vi "DPO4034 Fetch Measurement.vi"(7 "Destination Channel (1: Channel 2)":u16(ring)=1 items=["Channel 1", "Channel 2", "Channel 3", "Channel 4", "Math", "Reference 1", "Reference 2", "Reference 3", "Reference 4"], 8 "error in (no error)":errorcluster, 9 "Measurement Function (0: Period)":i32(ring) items=["Period", "Frequency", "Delay", "Rise Time", "Fall Time", "Positive Duty Cycle", "Negative Duty Cycle", "Positive Pulse Width", "Negative Pulse Width", "Burst Width", "Phase", "Positive Overshoot", "Negative Overshoot", "Vpp", "Amplitude", "Voltage High", "Voltage Low", "Voltage Max", "Voltage Min", "Voltage Mean", "Voltage Mean (cycle)", "Voltage RMS", "Voltage RMS (cycle)", "Area", "Cycle Area", "Positive Edge Count", "Negative Edge Count", "Positive Pulse Count", "Negative Pulse Count"], 10 "Channel (0: Channel 1)":u16(ring) items=["Channel 1", "Channel 2", "Channel 3", "Channel 4", "Math", "Reference 1", "Reference 2", "Reference 3", "Reference 4"], 11 "VISA resource name":refnum<visa-resource-name>) -> (0 "error out":errorcluster, 2 "Measurement Value":dbl, 3 "VISA resource name out":refnum<visa-resource-name>)   [LabVIEW 2012]
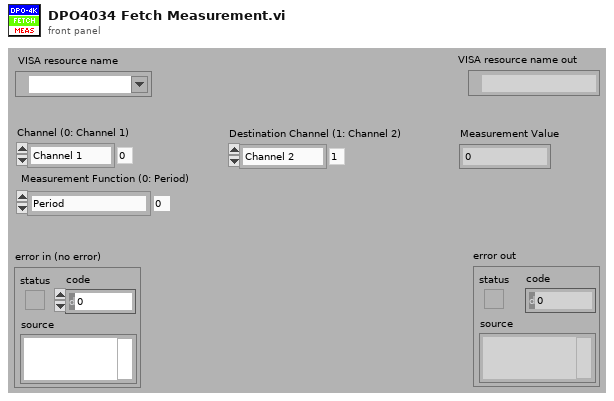
[diagram p1: front panel]
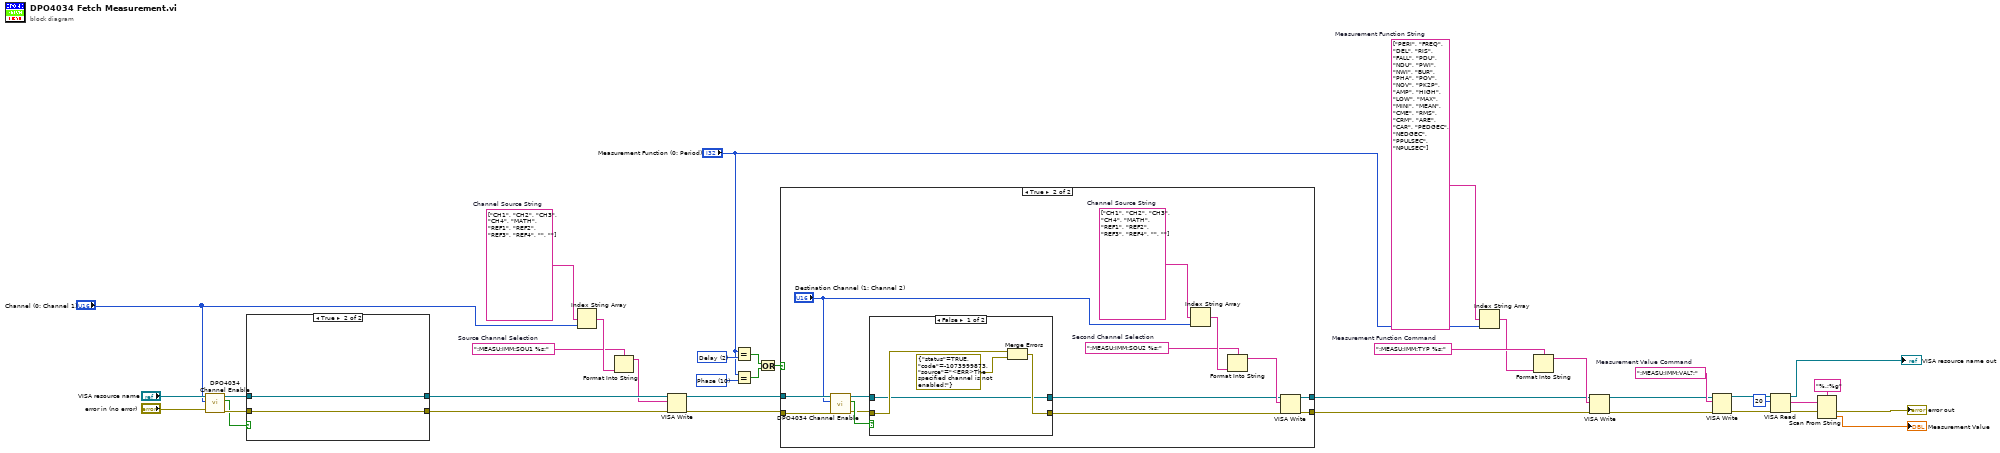
[diagram p0: block diagram]
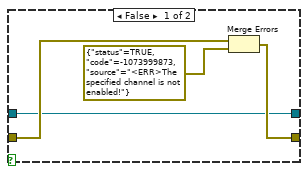
[diagram p2: hidden frame]
diagram:
  w12 = ":MEASU:IMM:SOU1 %s;"  # Source Channel Selection
  w11 = string[] ["CH1", "CH2", "CH3", "CH4", "MATH", "REF1", "REF2", "REF3", "REF4", "", ""]  # Channel Source String
  w26 = ":MEASU:IMM:VAL?;"  # Measurement Value Command
  w34 = u16 10 items=["Period", "Frequency", "Delay", "Rise Time", "Fall Time", "Positive Duty Cycle", "Negative Duty Cycle", "Positive Pulse Width", "Negative Pulse Width", "Burst Width", "Phase", "Positive Overshoot", "Negative Overshoot", "Pk-Pk", "Amplitude", "High", "Low", "Max", "Min", "Mean", "Cycle Mean", "RMS", "Cycle RMS", "Area", ""]
  w35 = u16 2 items=["Period", "Frequency", "Delay", "Rise Time", "Fall Time", "Positive Duty Cycle", "Negative Duty Cycle", "Positive Pulse Width", "Negative Pulse Width", "Burst Width", "Phase", "Positive Overshoot", "Negative Overshoot", "Pk-Pk", "Amplitude", "High", "Low", "Max", "Min", "Mean", "Cycle Mean", "RMS", "Cycle RMS", "Area", ""]
  w37 = ":MEASU:IMM:TYP %s;"  # Measurement Function Command
  w38 = string[] ["PERI", "FREQ", "DEL", "RIS", "FALL", "PDU", "NDU", "PWI", "NWI", "BUR", "PHA", "POV", "NOV", "PK2P", "AMP", "HIGH", "LOW", "MAX", "MINI", "MEAN", "CME", "RMS", "CRM", "ARE", "CAR", "PEDGEC", "NEDGEC", "PPULSEC", "NPULSEC"]  # Measurement Function String
  n1 = call "DPO4034 Channel Enable.vi"("error in (no error)"="error in (no error)", "Channel (0: Channel 1)"="Channel (0: Channel 1)", "VISA resource name"="VISA resource name") -> ("error out"=w3:errorcluster, "Enabled"=w1:bool, "VISA resource name out"=w2:refnum<visa-resource-name>)  [unwired: 6 in]
  n2 = case shown="True" w1 {
    tunnel: w2 -> [w39 w44]
    tunnel: w3 -> [w41 w43]
    tunnel: [w39 w44] -> w17
    tunnel: [w40 w43] -> w16
    frame False {
      n3 = Merge Errors(w41, errorcluster {"status"=TRUE, "code"=-1073999873, "source"="<ERR>The specified channel is not enabled!"} ("error out")) -> (w40:errorcluster)
    }
    frame True {
    }
  }
  n4 = Index String Array(1:"Channel (0: Channel 1)", 2:w11) -> (0:w13:string)  [unwired: 1 in]
  n5 = Format Into String(format string=w12, w13) -> (resulting string=w10:string)  [unwired: 2 in, 1 out]
  n6 = VISA Write(VISA resource name=w17, write buffer=w10, error in (no error)=w16) -> (VISA resource name out=w15:refnum<visa-resource-name>, error out=w14:errorcluster)  [unwired: 1 out]
  n7 = Equal?(x="Measurement Function (0: Period)", y=w35) -> (x = y?=w33:bool)
  n8 = Equal?(x="Measurement Function (0: Period)", y=w34) -> (x = y?=w32:bool)
  n9 = Or(x=w33, y=w32) -> (x .or. y?=w31:bool)
  n10 = case shown="True" w31 {
    tunnel: w15 -> [w46 w54]
    tunnel: w14 -> [w45 w53]
    tunnel: [w46 w57] -> w28
    tunnel: [w45 w56] -> w27
    frame False {
    }
    frame True {
      w58 = string[] ["CH1", "CH2", "CH3", "CH4", "MATH", "REF1", "REF2", "REF3", "REF4", "", ""]  # Channel Source String
      w59 = ":MEASU:IMM:SOU2 %s;"  # Second Channel Selection
      n11 = call "DPO4034 Channel Enable.vi"("error in (no error)"=w53, "Channel (0: Channel 1)"="Destination Channel (1: Channel 2)", "VISA resource name"=w54) -> ("error out"=w49:errorcluster, "Enabled"=w51:bool, "VISA resource name out"=w50:refnum<visa-resource-name>)  [unwired: 6 in]
      n12 = case shown="False" w51 {
        tunnel: w50 -> [w61 w66]
        tunnel: w49 -> [w63 w65]
        tunnel: [w61 w66] -> w48
        tunnel: [w62 w65] -> w47
        frame False {
          n13 = Merge Errors(w63, errorcluster {"status"=TRUE, "code"=-1073999873, "source"="<ERR>The specified channel is not enabled!"} ("error out")) -> (w62:errorcluster)
        }
        frame True {
        }
      }
      n14 = Index String Array(1:"Destination Channel (1: Channel 2)", 2:w58) -> (0:w60:string)  [unwired: 1 in]
      n15 = Format Into String(format string=w59, w60) -> (resulting string=w55:string)  [unwired: 2 in, 1 out]
      n16 = VISA Write(VISA resource name=w48, write buffer=w55, error in (no error)=w47) -> (VISA resource name out=w57:refnum<visa-resource-name>, error out=w56:errorcluster)  [unwired: 1 out]
    }
  }
  n17 = Index String Array(1:"Measurement Function (0: Period)", 2:w38) -> (0:w36:string)  [unwired: 1 in]
  n18 = Format Into String(format string=w37, w36) -> (resulting string=w30:string)  [unwired: 2 in, 1 out]
  n19 = VISA Write(VISA resource name=w28, write buffer=w30, error in (no error)=w27) -> (VISA resource name out=w19:refnum<visa-resource-name>, error out=w18:errorcluster)  [unwired: 1 out]
  n20 = VISA Write(VISA resource name=w19, write buffer=w26, error in (no error)=w18) -> (VISA resource name out=w25:refnum<visa-resource-name>, error out=w24:errorcluster)  [unwired: 1 out]
  n21 = VISA Read(VISA resource name=w25, byte count=u32 20, error in (no error)=w24) -> (VISA resource name out=→"VISA resource name out":refnum<visa-resource-name>, read buffer=w22:string, error out=w9:errorcluster)  [unwired: 1 out]
  n22 = Scan From String(format string="%.;%g", input string=w22, error in=w9) -> (error out=→"error out":errorcluster, output 1=→"Measurement Value":dbl)  [unwired: 2 in, 2 out]
